vi "SEA_9811_Select_FPGA.vi"(8 "error in (no error)":errorcluster, 11 "Item Ref in":T1 format="%.0x") -> (0 "error out":errorcluster, 3 "Item Ref out":T1 format="%.0x")   [LabVIEW 2015, in "AIT 429 System Explorer.lvlib"]
uses:
  AIT 429 System Explorer.lvlib
  <vilib>/NI Veristand/Custom Device API/Custom Device Item Ref.ctl
  <vilib>/NI Veristand/Custom Device API/Dependent File Optional Info.ctl
  Shared/Controls and Global/Global.vi
  <vilib>/NI Veristand/Custom Device API/Set Item Property (Dependent Node Pointer).vi
  <vilib>/NI Veristand/Custom Device API/Set Item Property (Dependent File).vi
  <vilib>/NI Veristand/Custom Device API/Set Item Property (Path).vi
  <vilib>/NI Veristand/Custom Device API/Set Item Property (String).vi
  <vilib>/NI Veristand/Custom Device API/Set Item Property (Boolean).vi
  <vilib>/NI VeriStand/Custom Device API/Custom Device API.lvlib
  Shared/ARINC 429 Shared.lvlib
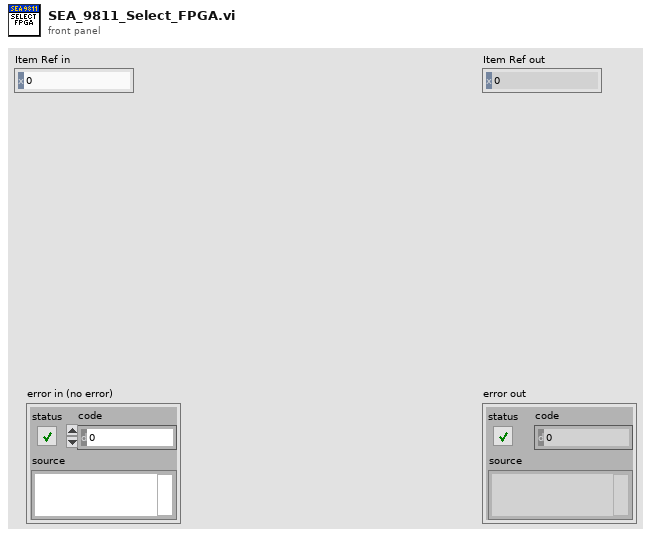
[diagram p1: front panel]
types:
  T1 = typedef "Custom Device API.lvlib/Custom Device Item Ref.ctl" = u64
  T2 = cluster{"RIO Device Address":string, "Bitfile Signature":string}
  T3 = typedef "Custom Device API.lvlib/Dependent File Optional Info.ctl" = cluster{"Version":string, "RTDestination":path, "ForceDownload":bool, "SupportedTarget":string, "MD5":string}
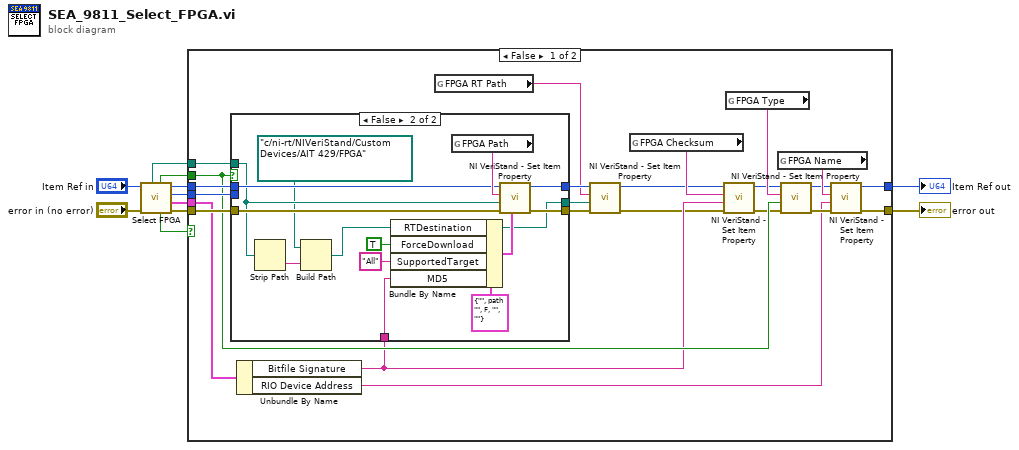
[diagram p0: block diagram]
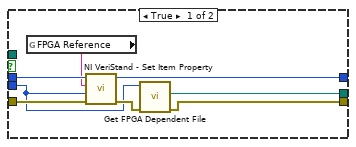
[diagram p2: hidden frame]
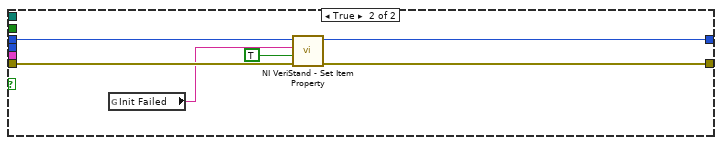
[diagram p3: hidden frame]
diagram:
  n1 = call "Select FPGA.vi"("error in"="error in (no error)", "Item Ref in"="Item Ref in") -> ("error out"=w8:errorcluster, "FPGA Info"=w7:T2, "FPGA Reference"=w6:T1, "Item Ref out"=w5:T1, "Cancelled?"=w9:bool, "VS FPGA?"=w4:bool, "Bitfile Path out"=w3:path)  [unwired: 3 in]
  n2 = case shown="False" w9 {
    tunnel: w6 -> [w34 _]
    tunnel: w8 -> [w33 w61]
    tunnel: w5 -> [w32 w62]
    tunnel: w7 -> [w31 _]
    tunnel: w4 -> [w30 _]
    tunnel: w3 -> [w29 _]
    tunnel: [w16 w60] -> w2
    tunnel: [w15 w57] -> w1
    frame False {
      n3 = Unbundle By Name(w31) -> ("Bitfile Signature"=w20:string, "RIO Device Address"=w21:string)
      n4 = case shown="False" w30 {
        tunnel: w34 -> [w39 _]
        tunnel: w33 -> [w41 w54]
        tunnel: w32 -> [w42 w55]
        tunnel: w29 -> [_ w51]
        tunnel: [w38 w53] -> w19
        tunnel: [w37 w52] -> w18
        tunnel: w20 -> [_ w44]
        tunnel: [w36 w43] -> w17
        frame True {
          n5 = global read "Global.vi" "FPGA Reference"() -> (w35:string)
          n6 = call-poly <vilib>:"NI VeriStand - Set Item Property.vi"("error in (no error)"=w41, "Dependent Node Ref"=w39, "Property Name"=w35, "Item Ref in"=w42) -> ("error out"=w40:errorcluster, "Item Ref out"=w37:T1)  [unwired: 5 in, 1 out]
          n7 = call "Get FPGA Dependent File.vi"("error in (no error)"=w40, "ID in"=w39) -> ("error out"=w38:errorcluster, "RT Path"=w36:path)  [unwired: 7 in, 1 out]
        }
        frame False {
          n8 = Strip Path(path=w51) -> (name=w50:string)  [unwired: 1 out]
          n9 = Build Path(base path=path "c:/ni-rt/NIVeriStand/Custom Devices/AIT 429/FPGA" ("RTDestination"), name or relative path=w50) -> (appended path=w43:path)
          n10 = Bundle By Name(cluster=T3 {"Version"="", "RTDestination"=path "", "ForceDownload"=FALSE, "SupportedTarget"="", "MD5"=""} ("OptionalInfo"), "RTDestination"=w43, "ForceDownload"=TRUE, "SupportedTarget"="All", "MD5"=w44) -> (w46:T3)
          n11 = global read "Global.vi" "FPGA Path"() -> (w56:string)
          n12 = call-poly <vilib>:"NI VeriStand - Set Item Property.vi"("OptionalInfo"=w46, "error in (no error)"=w54, "Path"=w51, "Property Name"=w56, "Item Ref in"=w55) -> ("error out"=w53:errorcluster, "Item Ref out"=w52:T1)  [unwired: 4 in, 1 out]
        }
      }
      n13 = global read "Global.vi" "FPGA RT Path"() -> (w14:string)
      n14 = call-poly <vilib>:"NI VeriStand - Set Item Property.vi"("error in (no error)"=w19, "Value"=w17, "Property Name"=w14, "Item Ref in"=w18) -> ("error out"=w13:errorcluster, "Item Ref out"=w12:T1)  [unwired: 5 in, 1 out]
      n15 = global read "Global.vi" "FPGA Checksum"() -> (w24:string)
      n16 = call-poly <vilib>:"NI VeriStand - Set Item Property.vi"("error in (no error)"=w13, "Value"=w20, "Property Name"=w24, "Item Ref in"=w12) -> ("error out"=w23:errorcluster, "Item Ref out"=w22:T1)  [unwired: 5 in, 1 out]
      n17 = global read "Global.vi" "FPGA Type"() -> (w25:string)
      n18 = global read "Global.vi" "FPGA Name"() -> (w28:string)
      n19 = call-poly <vilib>:"NI VeriStand - Set Item Property.vi"("error in (no error)"=w23, "Value"=w30, "Property Name"=w25, "Item Ref in"=w22) -> ("error out"=w26:errorcluster, "Item Ref out"=w27:T1)  [unwired: 5 in, 1 out]
      n20 = call-poly <vilib>:"NI VeriStand - Set Item Property.vi"("error in (no error)"=w26, "Value"=w21, "Property Name"=w28, "Item Ref in"=w27) -> ("error out"=w16:errorcluster, "Item Ref out"=w15:T1)  [unwired: 5 in, 1 out]
    }
    frame True {
      n21 = global read "Global.vi" "Init Failed"() -> (w58:string)
      n22 = call-poly <vilib>:"NI VeriStand - Set Item Property.vi"("error in (no error)"=w61, "Value"=TRUE, "Property Name"=w58, "Item Ref in"=w62) -> ("error out"=w60:errorcluster, "Item Ref out"=w57:T1)  [unwired: 5 in, 1 out]
    }
  }
  "error out" <- w2
  "Item Ref out" <- w1
